vi "Calculo_Velocidad.vi"(8 "error":dbl, 11 "Velocidad mm/s":dbl) -> (0 "V_min":dbl, 1 "V_max":dbl, 2 "Piñon 3":dbl, 3 "Piñon 1":dbl, 4 "V_f":dbl[][](array[numeric]), 6 "n_1":i32[](array[numeric]))   [LabVIEW 2013]
panel:
  out "h":dbl[][](array[numeric])
  out "Numeric 6":ext
  out "w_4":dbl[][](array[numeric])
  out "Numeric 4":ext
  out "Numeric 5":dbl
  out "g":dbl[](array[numeric])
  out "n_3":i32[](array[numeric])
  out "w_3s":dbl[][](array[numeric])
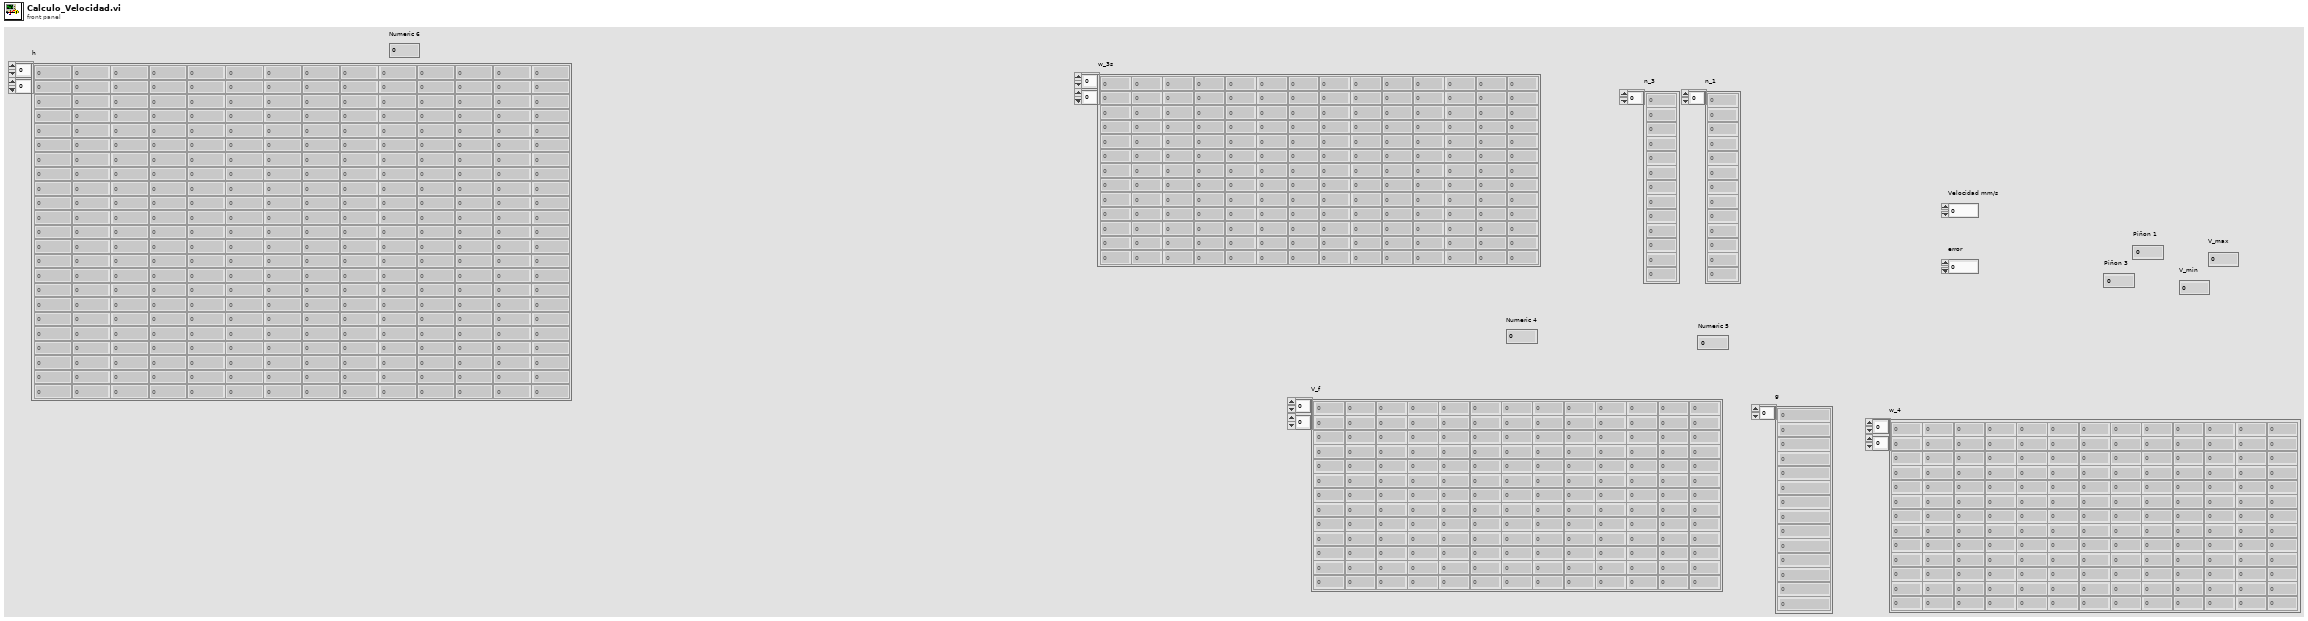
[diagram p1: front panel]
types:
  T1 = typedef "NI_Matrix.lvlib/RealMatrix.ctl" = dbl[][]
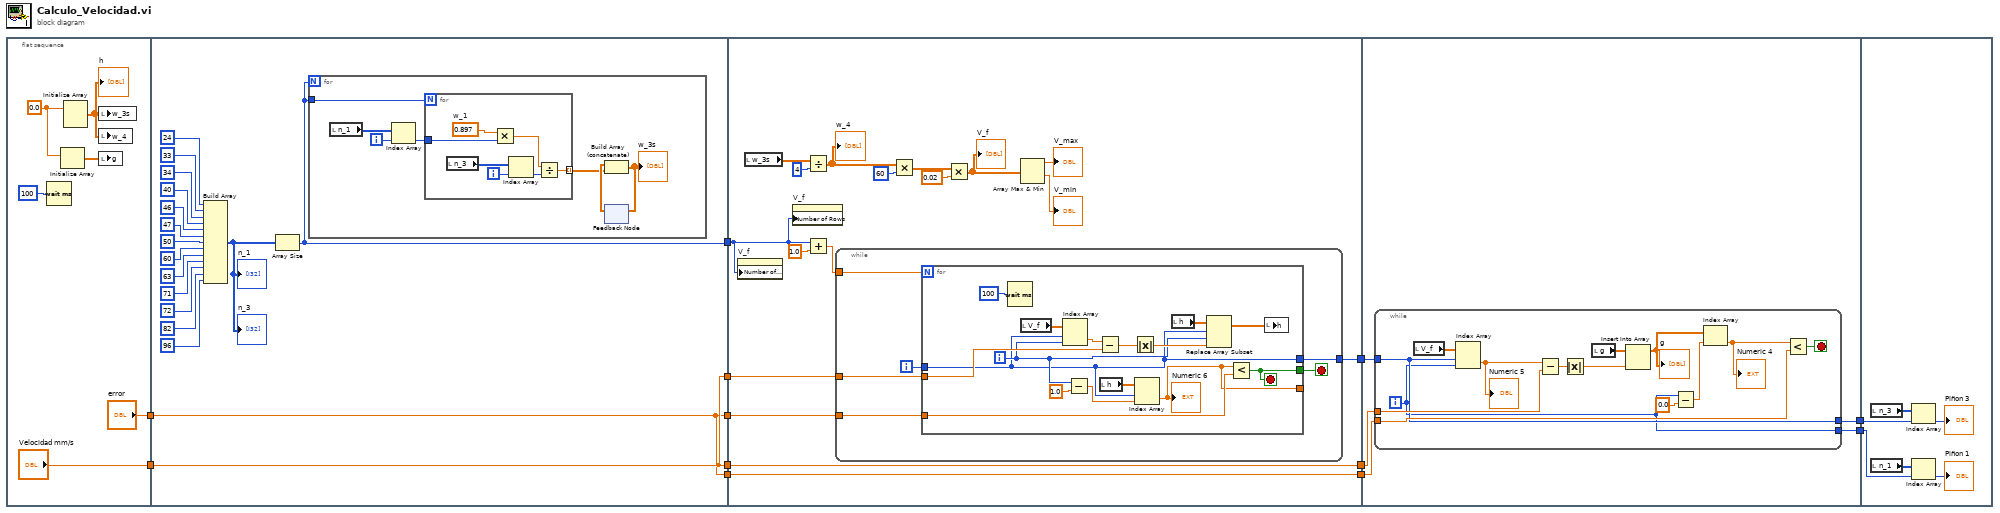
[diagram p0: block diagram]
diagram:
  n1 = flat-sequence {
    tunnel: ["Velocidad mm/s"] -> w10
    tunnel: ["error"] -> w8
    tunnel: [w19] -> w12
    tunnel: [w21] -> w11
    tunnel: w10 -> [w21]
    tunnel: [w21] -> w9
    tunnel: w8 -> [w20]
    tunnel: [w20] -> w7
    tunnel: [w20] -> w6
    tunnel: w12 -> [w50]
    tunnel: w11 -> [w57]
    tunnel: w9 -> [w54]
    tunnel: w7 -> [w56]
    tunnel: w6 -> [w55]
    tunnel: [w55] -> w4
    tunnel: [w54] -> w3
    tunnel: [w53] -> w2
    tunnel: [w89] -> w5
    tunnel: w4 -> [w93]
    tunnel: w3 -> [w92]
    tunnel: w2 -> [w91]
    tunnel: [w90] -> w1
    tunnel: w1 -> [w108]
    tunnel: w5 -> [w109]
    frame #0 {
      w14 = 0.0 ("element")
      n2 = Wait (ms)(milliseconds to wait=100) -> ()  [unwired: 1 out]
      n3 = Initialize Array(w14) -> (w15:dbl[])  [unwired: 1 in]
      n4 = Initialize Array(w14) -> (w13:dbl[][])  [unwired: 2 in]
      "h" <- w13
      n5 = local write "w_3s"(w13) -> ()
      n6 = local write "w_4"(w13) -> ()
      n7 = local write "g"(w15) -> ()
    }
    frame #1 {
      n8 = Build Array(24, 33, 34, 40, 46, 47, 50, 60, 63, 71, 72, 82, 96) -> (w34:i32[])
      "n_1" <- w34
      "n_3" <- w34
      n9 = Array Size(array=w34) -> (size(s)=w19:i32)
      n10 = for {
        N: w19 -> [_]
        tunnel: w19 -> [w42]
        i -> [w40]
        n11 = local read "n_1"() -> (w41:i32[])
        n12 = Index Array(array=w41, index=w40) -> (element=w39:i32)
        n13 = for {
          N: w42 -> [_]
          tunnel: w39 -> [w44]
          tunnel: [w43] -> w36 mode=indexing
          i -> [w48]
          w46 = 0.897  # w_1
          n14 = local read "n_3"() -> (w49:i32[])
          n15 = Multiply(x=w46, y=w44) -> (x*y=w47:dbl)
          n16 = Index Array(array=w49, index=w48) -> (element=w45:i32)
          n17 = Divide(x=w47, y=w45) -> (x/y=w43:dbl)
        }
        n18 = feedback #1() -> (w37:dbl[][])  [unwired: 1 in]
        n19 = Build Array (concatenate)(w37, w36) -> (w38:dbl[][])
        "w_3s" <- w38
        n20 = feedback-in #1(w38) -> ()
      }
    }
    frame #2 {
      n21 = property on="V_f" class="Arr (strict)"("Number of Columns"=w50) -> ()  [unwired: 2 in, 2 out]
      n22 = local read "w_3s"() -> (w62:dbl[][])
      n23 = property on="V_f" class="Arr (strict)"("Number of Rows"=w50) -> ()  [unwired: 2 in, 2 out]
      n24 = Divide(x=w62, y=4) -> (x/y=w60:dbl[][])
      "w_4" <- w60
      n25 = Add(x=w50, y=1.0) -> (x+y=w51:dbl)
      n26 = while {
        tunnel: w57 -> [w72]
        tunnel: w56 -> [w69]
        tunnel: [w70] -> w53
        tunnel: w51 -> [w67]
        i -> [w71]
        stop <- w68 stop-if-true
        n27 = for {
          N: w67 -> [_]
          tunnel: w72 -> [w86]
          tunnel: [w75] -> _
          tunnel: w71 -> [w77]
          tunnel: [w77] -> w70
          tunnel: w69 -> [w76]
          tunnel: [w74] -> w68
          i -> [w82]
          stop <- w74 stop-if-true
          n28 = Wait (ms)(milliseconds to wait=100) -> ()  [unwired: 1 out]
          n29 = local read "V_f"() -> (w88:dbl[][])
          n30 = Index Array(array=w88, index (row)=w77, index (col)=w82) -> (element=w87:dbl)
          n31 = Subtract(x=w82, y=1.0) -> (x-y=w78:dbl)
          n32 = Subtract(x=w87, y=w86) -> (x-y=w84:dbl)
          n33 = local read "h"() -> (w79:dbl[][])
          n34 = Absolute Value(x=w84) -> (abs(x)=w83:dbl)
          n35 = Index Array(array=w79, index (row)=w77, index (col)=w78) -> (element=w75:dbl)
          "Numeric 6" <- w75
          n36 = local read "h"() -> (w85:dbl[][])
          n37 = Replace Array Subset(array=w85, new element=w83, index (row)=w77, index (col)=w82) -> (w80:T1)
          n38 = Less?(x=w75, y=w76) -> (x < y?=w74:bool)
          n39 = local write "h"(w80) -> ()
        }
      }
      n40 = Multiply(x=w60, y=60) -> (x*y=w59:dbl[][])
      n41 = Multiply(x=w59, y=0.02) -> (x*y=w64:dbl[][])
      "V_f" <- w64
      n42 = Array Max & Min(array=w64) -> (max value=→"V_max":dbl, min value=→"V_min":dbl)  [unwired: 2 out]
    }
    frame #3 {
      n43 = while {
        tunnel: w92 -> [w105]
        tunnel: w93 -> [w104]
        tunnel: w91 -> [w101]
        tunnel: [w101] -> w90
        tunnel: [w98] -> w89
        i -> [w98]
        stop <- w99 stop-if-true
        n44 = local read "V_f"() -> (w107:dbl[][])
        n45 = Index Array(array=w107, index (row)=w101, index (col)=w98) -> (element=w94:dbl)
        "Numeric 5" <- w94
        n46 = Subtract(x=w94, y=w105) -> (x-y=w106:dbl)
        n47 = Absolute Value(x=w106) -> (abs(x)=w96:dbl)
        n48 = local read "g"() -> (w95:dbl[])
        n49 = Insert Into Array(array=w95, new element=w96) -> (w97:dbl[])  [unwired: 1 in]
        "g" <- w97
        n50 = Subtract(x=w98, y=0.0) -> (x-y=w103:dbl)
        n51 = Index Array(array=w97, index=w103) -> (element=w100:dbl)
        "Numeric 4" <- w100
        n52 = Less?(x=w100, y=w104) -> (x < y?=w99:bool)
      }
    }
    frame #4 {
      n53 = local read "n_3"() -> (w111:i32[])
      n54 = local read "n_1"() -> (w110:i32[])
      n55 = Index Array(array=w111, index=w108) -> (element=→"Piñon 3":i32)
      n56 = Index Array(array=w110, index=w109) -> (element=→"Piñon 1":i32)
    }
  }
